vi "triton_controller.vi"(9 "Increment":dbl=0.1, 10 "Numerical Argument":dbl, 11 "Command":T1(ring)=enum."Read Heater Voltage") -> (3 "Response":string)   [LabVIEW 2021]
panel:
  # "TRITON CONTROLLER"
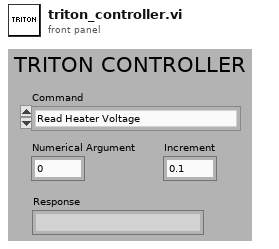
[diagram p1: front panel]
types:
  T1 = enum16{"Set Heater Voltage", "Read Heater Voltage", "Read Heater Current", "Read 1K Pot Temperature", "Read IVC Sorb Temperature", "Read Needle Valve Temperature", "Read Still Pressure", "Read Mixing Chamber Temperature", "Read STM RX Temperature", "Read STM CX Temperature", "Unstall Triton Loop", "Triton Stop", "Triton Stall Status"}
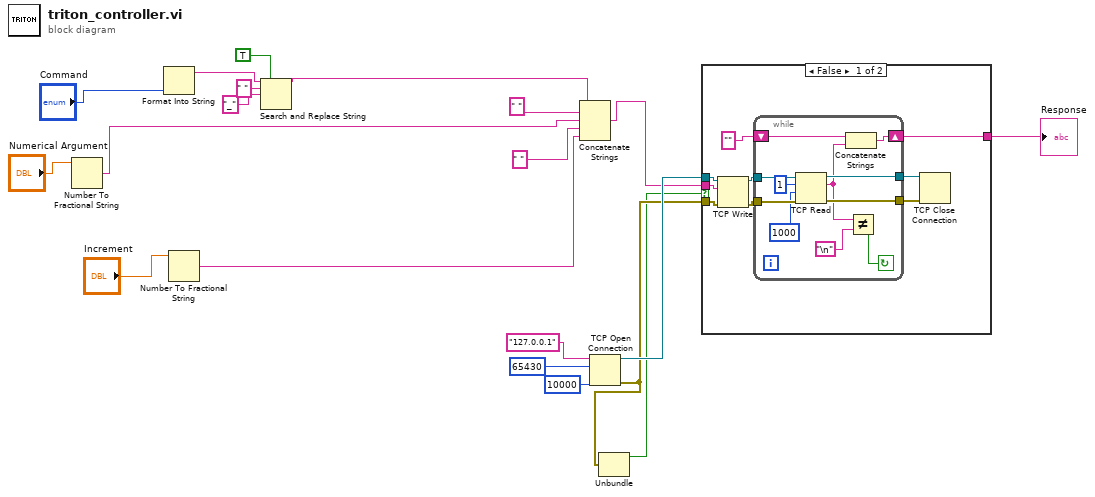
[diagram p0: block diagram]
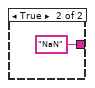
[diagram p2: hidden frame]
diagram:
  n1 = Number To Fractional String(number="Numerical Argument") -> (F-format string=w13:string)  [unwired: 3 in]
  n2 = Format Into String("Command") -> (resulting string=w12:string)  [unwired: 3 in, 1 out]
  n3 = Number To Fractional String(number="Increment") -> (F-format string=w1:string)  [unwired: 3 in]
  n4 = Search and Replace String(replace all?=TRUE ("replace all? (F)"), input string=w12, search string=" ", replace string="_" ("replace string (\"\")")) -> (result string=w11:string)  [unwired: 4 in, 3 out]
  n5 = Concatenate Strings(w11, " " ("string"), w13, " " ("string"), w1) -> (w17:string)
  n6 = TCP Open Connection(address="127.0.0.1", remote port or service name=u16 65430, timeout ms (60000)=10000) -> (connection ID=w18:refnum<k5>, error out=w7:errorcluster)  [unwired: 2 in]
  n7 = Unbundle(w7) -> ("status"=w6:bool)  [unwired: 2 out]
  n8 = case shown="False" w6 {
    tunnel: w18 -> [w29 _]
    tunnel: w7 -> [w28 _]
    tunnel: w17 -> [w22 _]
    tunnel: [w21 "NaN" ("string")] -> w5
    frame False {
      n9 = TCP Write(connection ID=w29, data in=w22, error in (no error)=w28) -> (connection ID out=w26:refnum<k5>, error out=w27:errorcluster)  [unwired: 1 in, 1 out]
      n10 = while {
        tunnel: w27 -> [w40]
        tunnel: w26 -> [w39]
        tunnel: [w38] -> w25
        tunnel: [w37] -> w24
        shift-right: [w33] -> w21
        shift-left: "" ("string") -> [w34]
        stop <- w32 continue-if-true
        n11 = TCP Read(connection ID=w39, bytes to read=1, error in (no error)=w40, 9:1000 ("timeout ms (25000)")) -> (connection ID out=w37:refnum<k5>, data out=w31:string, error out=w38:errorcluster)  [unwired: 1 in]
        n12 = Concatenate Strings(w34, w31) -> (w33:string)
        n13 = Not Equal?(x=w31, y="\n") -> (x != y?=w32:bool)
      }
      n14 = TCP Close Connection(connection ID=w24, error in (no error)=w25) -> ()  [unwired: 1 in, 2 out]
    }
    frame True {
    }
  }
  "Response" <- w5
